vi "Step Mode - Read DC Voltage Setting.vi"(8 "error in (no error)":errorcluster, 11 "VISA resource name":refnum<visa-resource-name>) -> (0 "error out":errorcluster, 2 "DC Voltage":dbl, 3 "VISA resource name out":refnum<visa-resource-name>)   [LabVIEW 2014, in "Associated Power Technologies 8500 Series.lvlib"]
doc: "Get the setting of basic DC voltage."
uses:
  <instrlib>/Associated Power Technologies 8500 Series/Associated Power Technologies 8500 Series.lvlib
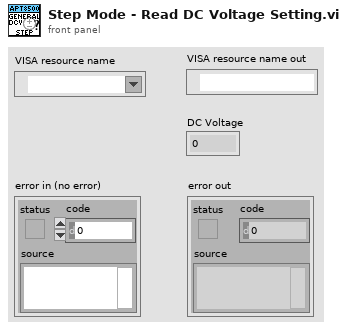
[diagram p1: front panel]
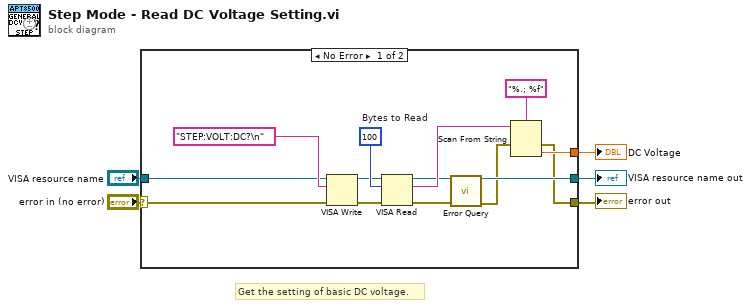
[diagram p0: block diagram]
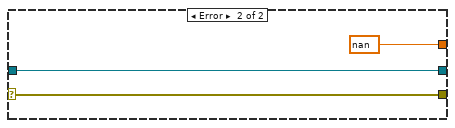
[diagram p2: hidden frame]
diagram:
  # "Get the setting of basic DC voltage."
  n1 = case shown="No Error" "error in (no error)" {
    selector: "error in (no error)" -> [w15 w22]
    tunnel: [w6 w22] -> w3
    tunnel: [w10 w21] -> w2
    tunnel: "VISA resource name" -> [w14 w21]
    tunnel: [w11 nan] -> w1
    frame No Error {
      w19 = u32 100  # Bytes to Read
      n2 = VISA Write(VISA resource name=w14, write buffer="STEP:VOLT:DC?\n", error in (no error)=w15) -> (VISA resource name out=w17:refnum<visa-resource-name>, error out=w18:errorcluster)  [unwired: 1 out]
      n3 = VISA Read(VISA resource name=w17, byte count=w19, error in (no error)=w18) -> (VISA resource name out=w9:refnum<visa-resource-name>, read buffer=w13:string, error out=w8:errorcluster)  [unwired: 1 out]
      n4 = call <instrlib>:"Error Query.vi"("VISA resource name"=w9, "error in (no error)"=w8) -> ("VISA resource name out"=w10:refnum<visa-resource-name>, "error out"=w7:errorcluster)  [unwired: 10 in, 2 out]
      n5 = Scan From String(format string="%.; %f", input string=w13, error in=w7) -> (error out=w6:errorcluster, output 1=w11:dbl)  [unwired: 2 in, 2 out]
    }
    frame Error {
    }
  }
  "VISA resource name out" <- w2
  "error out" <- w3
  "DC Voltage" <- w1
